vi "HP34970A Conf Scan List.vi"(6 "Scan List(empty)":string, 8 "error in (no error)":errorcluster, 9 "Check Parameter(0:Scan Lis)":enum16{"Scan List", "Scan Size"}(ring), 10 "Set/Check (F:Set)":bool, 11 "VISA session":refnum<visa-resource-name>) -> (0 "error out":errorcluster, 2 "Configuration?":string, 3 "dup VISA session":refnum<visa-resource-name>)   [LabVIEW 2020]
doc: "This VI lets you configure or check the scan list."
panel:
  # "Check\nSet"
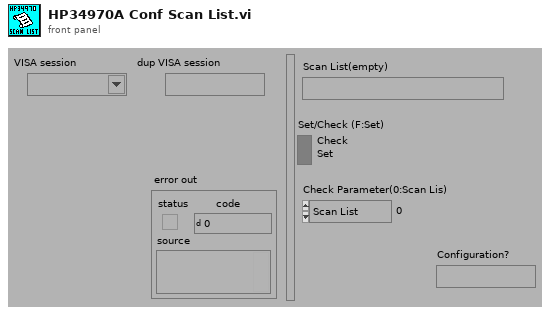
[diagram p1: front panel]
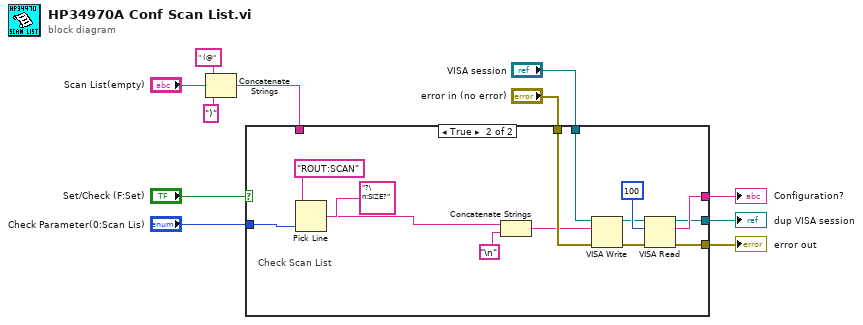
[diagram p0: block diagram]
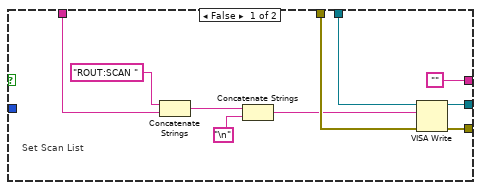
[diagram p2: hidden frame]
diagram:
  n1 = Concatenate Strings(" (@", "Scan List(empty)", ")") -> (w6:string)
  n2 = case shown="True" "Set/Check (F:Set)" {
    tunnel: [w17 w35] -> w10
    tunnel: [w18 w32] -> w11
    tunnel: w6 -> [w15 _]
    tunnel: ["" w33] -> w5
    tunnel: "VISA session" -> [w20 w31]
    tunnel: "error in (no error)" -> [w19 w30]
    tunnel: "Check Parameter(0:Scan Lis)" -> [_ w25]
    frame False {
      # "Set Scan List"
      n3 = Concatenate Strings("ROUT:SCAN ", w15) -> (w13:string)
      n4 = Concatenate Strings(w13, "\n") -> (w12:string)
      n5 = VISA Write(VISA resource name=w20, write buffer=w12, error in (no error)=w19) -> (VISA resource name out=w18:refnum<visa-resource-name>, error out=w17:errorcluster)  [unwired: 1 out]
    }
    frame True {
      # "Check Scan List"
      n6 = Pick Line(string ("")="ROUT:SCAN", multi-line string="?\n:SIZE?", line index=w25) -> (output string=w23:string)
      n7 = Concatenate Strings(w23, "\n") -> (w22:string)
      n8 = VISA Write(VISA resource name=w31, write buffer=w22, error in (no error)=w30) -> (VISA resource name out=w29:refnum<visa-resource-name>, error out=w28:errorcluster)  [unwired: 1 out]
      n9 = VISA Read(VISA resource name=w29, byte count=u32 100 ("byte count (0)"), error in (no error)=w28) -> (VISA resource name out=w32:refnum<visa-resource-name>, read buffer=w33:string, error out=w35:errorcluster)  [unwired: 1 out]
    }
  }
  "dup VISA session" <- w11
  "error out" <- w10
  "Configuration?" <- w5
